vi "packages versions global.vi"() -> ()   [LabVIEW 2018, in "LV2Julia_core.lvlib"]
uses:
  LV2Julia_core.lvlib
  VersionNumber.ctl
panel:
  in  "packages versions":T2={"LV_v"={"major"=0, "minor"=2, "patch"=2}, "LVServer_current"={"major"=0, "minor"=2, "patch"=2}, "LVServer_min"={"major"=0, "minor"=2, "patch"=2}}
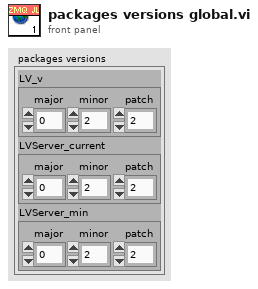
[diagram p1: front panel]
types:
  T1 = typedef "LV2Julia_core.lvlib/VersionNumber.ctl" = cluster{"major":u16, "minor":u16, "patch":u16}
  T2 = cluster{"LV_v":T1, "LVServer_current":T1, "LVServer_min":T1}
diagram:
